vi "save data to main file.vi"(0 "dont save":bool, 1 "save data":bool, 7 "exp exec in":T1, 11 "primary":bool) -> (3 "results":dbl[][](array[numeric]) format="%#_3e", 4 "data file path":path, 8 "exp exec out":T1, 14 "Experimental Sequence":T7, 15 "stop":bool)   [LabVIEW 2019]
doc: "This is a Bug C(T) subVI.\n\nIt saves the data to existing data file at the conclusion of the experiment.\n\nPaul K Dixon\nP3600\nCSUSB Physics"
uses:
  typedefs/PID exec cluster.ctl
  typedefs/data file info.ctl
  typedefs/bug temp file info.ctl
  typedefs/exp seq cluster.ctl
  typedefs/wvfm acq params.ctl
  typedefs/bug meas status.ctl
  typedefs/exp sequence.ctl
  globals/Bug globals.vi
  <vilib>/Utility/file.llb/Write Delimited Spreadsheet (DBL).vi
panel:
  in  "Header":string="This is a C(T) experiment being done in Physics 3600.\nIt records the decay response of an RC circuit where the capacitance is a strong function of temperature." caption="Header Comments"
  in  "String":string="waveform params\tn meas\tindex\ttemp (C)\ttime (S)\tcapacitance (F)\tnormalized waveforms"
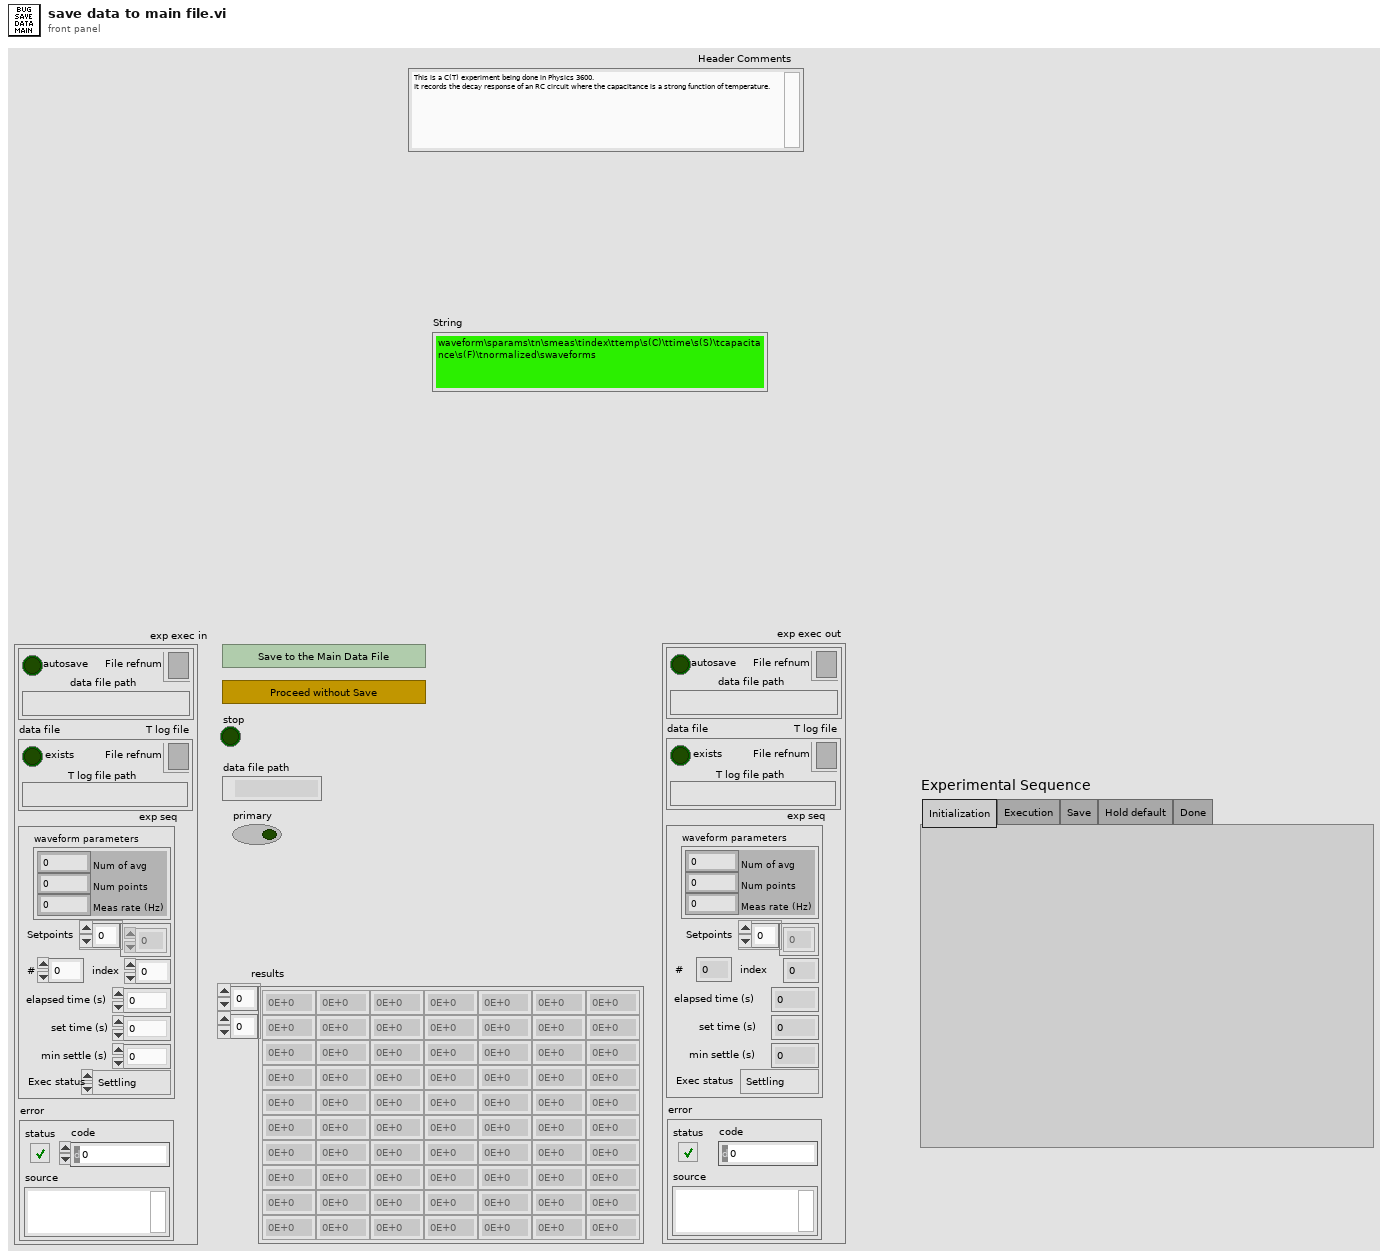
[diagram p1: front panel]
types:
  T1 = typedef "PID exec cluster.ctl" = cluster{"data file":T2, "T log file":T3, "exp seq":T4, "error":errorcluster}
  T2 = typedef "data file info.ctl" = cluster{"autosave":bool, "File refnum":refnum<file>, "data file path":path}
  T3 = typedef "bug temp file info.ctl" = cluster{"File refnum":refnum<file>, "T log file path":path, "exists":bool}
  T4 = typedef "exp seq cluster.ctl" = cluster{"wave params":T5, "Setpoints":dbl[], "#":i32, "index":i32, "elapsed time (s)":dbl, "set time (s)":dbl, "min settle (s)":dbl, " Exec Status":T6}
  T5 = typedef "wvfm acq params.ctl" = cluster{"Num of avg":i32, "Num points":i32, "Meas rate (Hz)":dbl}
  T6 = typedef "bug meas status.ctl" = enum32{"Settling", "Measuring", "Holding", "Exit"}
  T7 = typedef "exp sequence.ctl" = enum32{"Initialization", "Execution", "Save", "Hold default", "Done"}
  T8 = typedef "result.ctl" = cluster{"Temp (C)":dbl, "RC Fit":T9, "wave":waveform(dbl), "Time (s)":dbl}
  T9 = typedef "cap fit params.ctl" = cluster{"Resistance (Ohms)":dbl, "Est Time constant (s)":dbl, "Est Capacitance (F)":dbl}
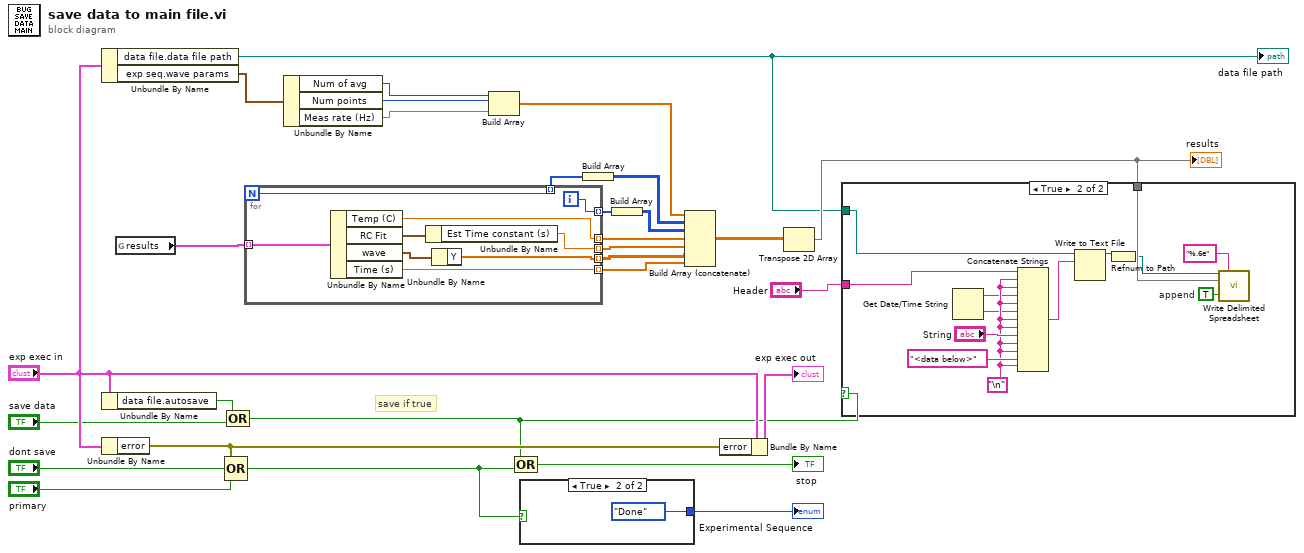
[diagram p0: block diagram]
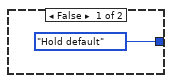
[diagram p3: hidden frame]
diagram:
  # "save if true"
  n1 = Unbundle By Name("exp exec in") -> ("data file.data file path"=w1:path, "exp seq.wave params"=w18:T5)
  "data file path" <- w1
  n2 = Unbundle By Name("exp exec in") -> ("data file.autosave"=w21:bool)
  n3 = Unbundle By Name("exp exec in") -> ("error"=w20:errorcluster)
  n4 = global read "Bug globals.vi" "results"() -> (w19:T8[])
  n5 = Compound Arithmetic op=OR(w20, "dont save", "primary") -> (w23:bool)
  n6 = Compound Arithmetic op=OR(w21, "save data") -> (w4:bool)
  n7 = for {
    N -> [w36]
    tunnel: w19 -> [w38] mode=indexing
    tunnel: [w36] -> w14 mode=indexing
    tunnel: [w35] -> w13 mode=indexing
    tunnel: [w34] -> w9 mode=indexing
    tunnel: [w33] -> w8 mode=indexing
    tunnel: [w32] -> w7 mode=indexing
    tunnel: [w30] -> w6 mode=indexing
    i -> [w35]
    n8 = Unbundle By Name(w38) -> ("Temp (C)"=w34:dbl, "RC Fit"=w37:T9, "wave"=w31:waveform(dbl), "Time (s)"=w32:dbl)
    n9 = Unbundle By Name(w37) -> ("Est Time constant (s)"=w33:dbl)
    n10 = Unbundle By Name(w31) -> ("Y"=w30:dbl[])
  }
  n11 = Unbundle By Name(w18) -> ("Num of avg"=w17:i32, "Num points"=w16:i32, "Meas rate (Hz)"=w15:dbl)
  n12 = Build Array(w17, w16, w15) -> (w10:dbl[])
  n13 = Compound Arithmetic op=OR(w4, w23) -> (→"stop":bool)
  n14 = case shown="True" w23 {
    tunnel: [exp_sequence."Hold default" ("Experimental Sequence") exp_sequence."Done" ("Experimental Sequence")] -> w28
    frame False {
    }
    frame True {
    }
  }
  "Experimental Sequence" <- w28
  n15 = Build Array(w14) -> (w12:i32[][])
  n16 = Build Array(w13) -> (w11:i32[][])
  n17 = Build Array (concatenate)(w10, w12, w11, w9, w8, w6, w7) -> (w5:dbl[][])
  n18 = Bundle By Name(cluster="exp exec in", "error"=w20) -> (→"exp exec out":T1)
  n19 = Transpose 2D Array(2D array=w5) -> (transposed array=w2:dbl[][])
  "results" <- w2
  n20 = case shown="True" w4 {
    tunnel: "Header" -> [_ w46]
    tunnel: w2 -> [_ w45]
    tunnel: w1 -> [_ w44]
    frame False {
    }
    frame True {
      w49 = "\n"
      w52 = TRUE  # append
      n21 = Get Date/Time String() -> (date string=w47:string, time string=w48:string)  [unwired: 3 in]
      n22 = Concatenate Strings(w46, w49, w49, w47, w49, w48, w49, w49, "String", w49, w49, "<data below>", w49) -> (w43:string)
      n23 = Write to Text File(file (use dialog)=w44, text=w43) -> (refnum out=w42:refnum<file>)  [unwired: 1 in, 3 out]
      n24 = Refnum to Path(1:w42) -> (0:w41:path)
      n25 = call-poly <vilib>:"Write Delimited Spreadsheet.vi"("file path (dialog if empty)"=w41, "format (%.3f)"="%.6e", "2D data"=w45, "append to file? (new file:F)"=w52) -> ()  [unwired: 10 in, 2 out]
    }
  }
